vi "digitalWrite.vi"(8 "Error In":errorcluster, 10 "value":bool, 11 "Digital Pin":T1 items=["D0"=0, "D1"=1, "D2"=2, "D3"=3, "D4"=4, "D5"=5, "D6"=6, "D7"=7, "D8"=8, "D9"=9, "D10"=10, "D11"=11, "D12"=12, "D13"=13, "D14"=14, "D15"=15, "LED_BUILTIN"=1001]) -> (0 "Error Out":errorcluster, 3 "resulting string":string)   [LabVIEW 2014]
uses:
  ctl/digitalPin.ctl
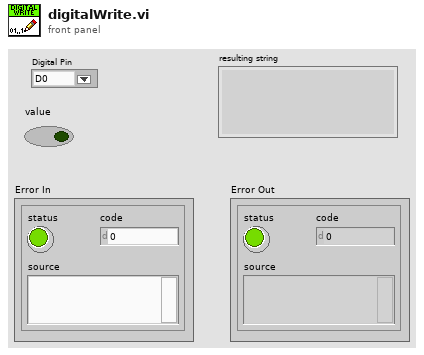
[diagram p1: front panel]
types:
  T1 = typedef "digitalPin.ctl" = u16
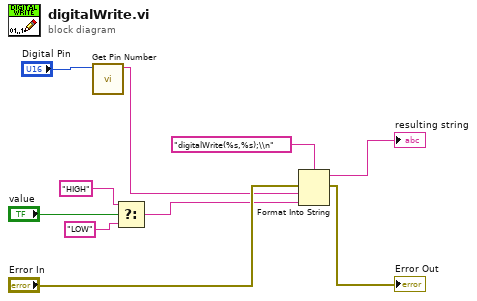
[diagram p0: block diagram]
diagram:
  n1 = call "Get Pin Number.vi"("pin number"="Digital Pin") -> ("String"=w5:string)  [unwired: 10 in]
  n2 = Select(t="HIGH", s="value", f="LOW") -> (s? t:f=w4:string)
  n3 = Format Into String(format string="digitalWrite(%s,%s);\\n", error in="Error In", w5, w4) -> (resulting string=→"resulting string":string, error out=→"Error Out":errorcluster)  [unwired: 1 in]
